vi "Get Config File Path.vi"(8 "error in (no error)":errorcluster, 10 "SaveDefault=false":bool, 11 "Settings":T1 {"Hardware Configuration"."Lasers Configuration"."SettingValues"."785 Power" format="%.1f"; "Hardware Configuration"."Lasers Configuration"."SettingValues"."647 Power" format="%.1f"; "Hardware Configuration"."Lasers Configuration"."SettingValues"."561 Power" format="%.1f"; "Hardware Configuration"."Lasers Configuration"."SettingValues"."532 Power" format="%.1f"; "Hardware Configuration"."Lasers Configuration"."SettingValues"."488 Power" format="%.1f"; "Hardware Configuration"."Lasers Configuration"."SettingValues"."405 Power" format="%.1f"}) -> (0 "error out":errorcluster, 3 "XML File Path":path)   [LabVIEW 2019, in "Settings.lvlib"]
doc: "Get the path to the Settings XML file. This is done using the Application Directory function. For more information on how Application Directory calculates its path, right-click the function and choose Help."
uses:
  Settings.lvlib
  Settings.ctl
  HardwareAdapter/Support/Hardware Configuration.ctl
  HardwareAdapter/Support/Camera Configuration.ctl
  D:/SDK/PMQI-LabViewSamples/Examples/Dependencies/PVCamNET.dll
  <vilib>/userdefined/High Color/IMAQdx.ctl
  E:/DevHardSoftware/MMicroscopy/HardwareAdapter/Lasers/Dependencies/Oxxius_Boxx.dll
  HardwareAdapter/Lasers/Dependencies/Oxxius_Boxx.dll
  Logging/Logging Configuration.ctl
  controls/UI Configuration.ctl
  controls/CallBack Refs.ctl
  Logging/Logging.lvlib
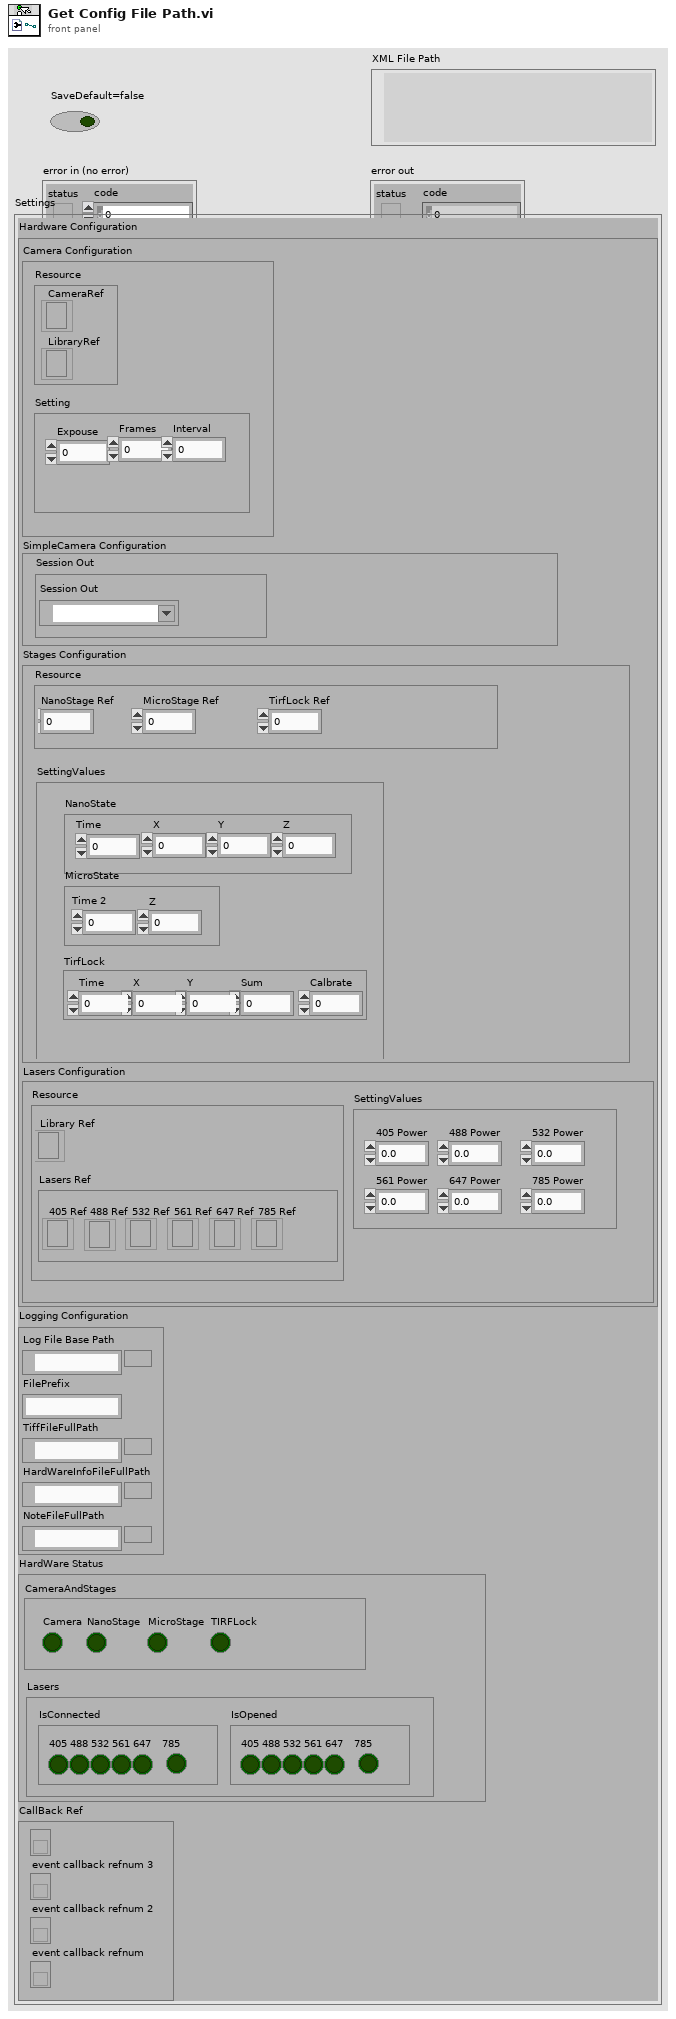
[diagram p1: front panel]
types:
  T1 = typedef "Settings.lvlib/Settings.ctl" = cluster{"Hardware Configuration":T2, "Logging Configuration":T5, "HardWare Status":cluster{"CameraAndStages":T6, "Lasers":cluster{"IsConnected":cluster{"405":bool, "488":bool, "532":bool, "561":bool, "647":bool, "785":bool}, "IsOpened":cluster{"405":bool, "488":bool, "532":bool, "561":bool, "647":bool, "785":bool}}}, "CallBack Ref":T7}
  T2 = typedef "Hardware Configuration.ctl" = cluster{"Camera Configuration":T3, "SimpleCamera Configuration":cluster{"Resource":cluster{"Session Out":T4}}, "Stages Configuration":cluster{"Resource":cluster{"NanoStage Ref":i32, "MicroStage Ref":i32, "TirfLock Ref":i32}, "SettingValues":cluster{"NanoState":cluster{"Time":dbl, "X":dbl, "Y":dbl, "Z":dbl}, "MicroState":cluster{"Time 2":dbl, "Z":dbl}, "TirfLock":cluster{"Time":dbl, "X":dbl, "Y":dbl, "Sum":dbl, "Calbrate":dbl}}}, "Lasers Configuration":cluster{"SettingValues":cluster{"405 Power":sgl, "488 Power":sgl, "532 Power":sgl, "561 Power":sgl, "647 Power":sgl, "785 Power":sgl}, "Resource":cluster{"Library Ref":refnum<k24>, "Lasers Ref":cluster{"405 Ref":refnum<k24>, "488 Ref":refnum<k24>, "532 Ref":refnum<k24>, "561 Ref":refnum<k24>, "647 Ref":refnum<k24>, "785 Ref":refnum<k24>}}}}
  T3 = typedef "Camera Configuration.ctl" = cluster{"Resource":cluster{"CameraRef":refnum<k24>, "LibraryRef":refnum<k24>}, "Setting":cluster{"Expouse":dbl, "Frames":dbl, "Interval":dbl}}
  T4 = typedef "IMAQdx.ctl" = refnum<k21>
  T5 = typedef "Logging.lvlib/Logging Configuration.ctl" = cluster{"Log File Base Path":path, "FilePrefix":string, "TiffFileFullPath":path, "HardWareInfoFileFullPath":path, "NoteFileFullPath":path}
  T6 = typedef "UI Configuration.ctl" = cluster{"Camera":bool, "NanoStage":bool, "MicroStage":bool, "TIRFLock":bool}
  T7 = typedef "CallBack Refs.ctl" = cluster{"event callback refnum":refnum<k27>, "event callback refnum 2":refnum<k27>, "event callback refnum 3":refnum<k27>, "event callback refnum 4":refnum<k27>}
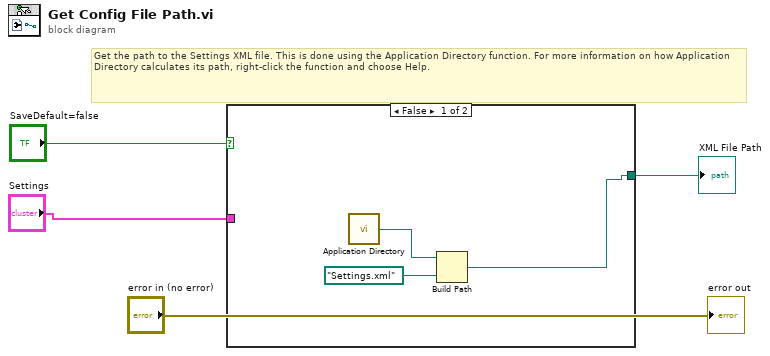
[diagram p0: block diagram]
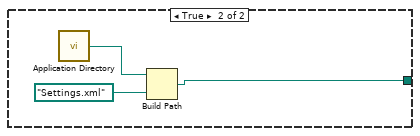
[diagram p2: hidden frame]
diagram:
  # "Get the path to the Settings XML file. This is done using the Application Directory function. For more information on how Application Directory calculates its path, right-click the function and choose Help."
  n1 = case shown="False" "SaveDefault=false" {
    tunnel: "Settings" -> [_ _]
    tunnel: [w5 w8] -> w1
    frame False {
      n2 = call <vilib>:"Application Directory.vi"() -> ("Application Directory"=w6:path)
      n3 = Build Path(base path=w6, name or relative path=path "Settings.xml" ("string")) -> (appended path=w5:path)
    }
    frame True {
      n4 = call <vilib>:"Application Directory.vi"() -> ("Application Directory"=w9:path)
      n5 = Build Path(base path=w9, name or relative path=path "Settings.xml" ("string")) -> (appended path=w8:path)
    }
  }
  "XML File Path" <- w1
  "error out" <- "error in (no error)"
